vi "Start File.vi"(8 "error in (no error)":errorcluster, 11 "Pulse Echo in":refnum<class "IV.lvclass">) -> (0 "error out":errorcluster, 2 "File Path":path, 3 "Pulse Echo out":refnum<class "IV.lvclass">)   [LabVIEW 2021, in "IV.lvclass"]
uses:
  IV.lvclass
  Libraries/File/File Class/File.lvclass
  IV.lvclass/IV.ctl
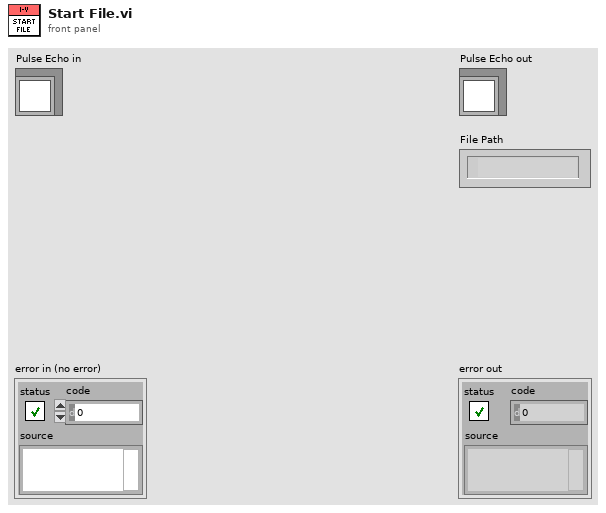
[diagram p1: front panel]
types:
  T1 = typedef "IV Config.ctl" = cluster{"Start current":dbl, "End current":dbl, "Current step":dbl, "Step time":dbl}
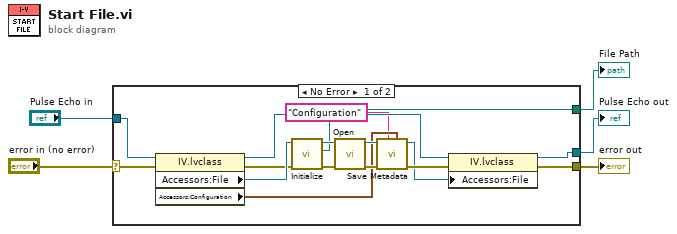
[diagram p0: block diagram]
diagram:
  n1 = case shown="No Error" "error in (no error)" {
    selector: "error in (no error)" -> [w21 w23]
    tunnel: [w11 w23] -> w4
    tunnel: [w9 w22] -> w2
    tunnel: "Pulse Echo in" -> [w20 w22]
    tunnel: [w7 _] -> w1
    frame No Error {
      n2 = property class="IV.lvclass"(reference=w20, error in=w21) -> (reference out=w10:refnum<class "IV.lvclass">, error out=w16:errorcluster, "Accessors:File"=w17:refnum<class "File.lvclass">, "Accessors:Configuration"=w13:T1)
      n3 = call-dynamic "Initialize.vi"("error in (no error)"=w16, "File in"=w17) -> ("error out"=w19:errorcluster, "File Path"=w7:path, "File out"=w18:refnum<class "File.lvclass">)  [unwired: 7 in]
      n4 = call-dynamic "Open.vi"("error in (no error)"=w19, "File in"=w18) -> ("error out"=w15:errorcluster, "File out"=w14:refnum<class "File.lvclass">)  [unwired: 7 in, 1 out]
      n5 = call-dynamic "Save Metadata.vi"("property value"=w13, "name"="Configuration", "error in (no error)"=w15, "File in"=w14) -> ("error out"=w12:errorcluster, "File out"=w8:refnum<class "File.lvclass">)  [unwired: 4 in, 2 out]
      n6 = property class="IV.lvclass"(reference=w10, error in=w12, "Accessors:File"=w8) -> (reference out=w9:refnum<class "IV.lvclass">, error out=w11:errorcluster)
    }
    frame Error {
    }
  }
  "error out" <- w4
  "Pulse Echo out" <- w2
  "File Path" <- w1
